vi "Acquisition & Generation (Init Memory-clock) test - Copia.vi"   [LabVIEW 2014]
uses:
  <vilib>/Platform/TimedLoop/XDataNode/timing_clust.ctl
  <vilib>/Platform/TimedLoop/XDataNode/nitl_modes.ctl
  <vilib>/Platform/TimedLoop/XDataNode/wakeup.ctl
  <vilib>/rvi/Emulation/niFpgaSctlEmulationGetInTimedLoop.vi
  <vilib>/rvi/Emulation/niFpgaEmulationReportErrorSimple.vi
  <vilib>/rvi/Emulation/niFpgaGetClockAttributes.vi
  <vilib>/rvi/Emulation/niFpgaCriticalErrorInLSC.vi
  <vilib>/rvi/Memory/Memory_Emulation/nirvimemoryFastEmulation.vi
  <vilib>/rvi/Memory/Memory_Emulation/nirvimemoryEmulation.vi
  <vilib>/rvi/Emulation/niFpgaEmulationIsFPGAContextNoSignature.vi
  <vilib>/rvi/DataTransferAndStorage/Container/Common/niFpgaContainerGetUniqueNameForEmu.vi
  <vilib>/rvi/Emulation/niFpgaProcessEmulError.vi
  <vilib>/rvi/errors/nirviReportUnexpectedCaseInternalError (U32).vi
  <vilib>/rvi/errors/niFpgaSetErrorForExecOnDevCompSimple.vi
  <vilib>/rvi/eio/common/nirviEmuReportErrorAndStop.vi
  <vilib>/rvi/FIFO/Fifo_Resource/nirvififoEmulationSetSize.vi
  <vilib>/rvi/FIFO/Fifo_Resource/nirviFifoEmulationQueueMgr.vi
  <instcachedir>/0/nirviFifoEmulationQueueMgr_E5CAEC123FF24DC58D834DCA3CDAA9B5.lvgen/nirviFifoEmulationQueueMgr_E5CAEC123FF24DC58D834DCA3CDAA9B5_010.vi
  <vilib>/rvi/FIFO/Fifo_Resource/nirvififoEmulationDetermineInputValidOut.vi
  <vilib>/rvi/FIFO/Fifo_Resource/nirvififoEmulationCreateLock.vi
  <vilib>/rvi/FIFO/Fifo_Resource/nirvififoEmulationObtainLock.vi
  <vilib>/rvi/FIFO/Fifo_Resource/nirvififoEmulationReleaseLock.vi
  <vilib>/rvi/occurrence/nirviWaitOnOccurrenceBase.vi
  <vilib>/rvi/errors/nirviReportUnexpectedCaseInternalError.vi
  <vilib>/rvi/eio/common/nirviEmuTemplateMethod_errors.vi
  <vilib>/rvi/interface/RandomDataEmulation/niFpgaRandomDataHandleErrors.vi
  <vilib>/Platform/TimedLoop/XDataNode/XDataNode.xnode
  <vilib>/rvi/DataTransferAndStorage/Container/XNode/niFpgaContainer.xnode
  <vilib>/rvi/FIFO/Fifo_Resource/nirvififoEmulationWrite.vi
  <vilib>/rvi/FIFO/Fifo_Resource/nirvififoEmulationRead.vi
  <vilib>/eio/EIOMethodNode/EIOMethodNode.xnode
  <vilib>/rvi/interface/RandomDataEmulation/nirviRandomDataFpgaReadWriteTemplate.vi
  <vilib>/Platform/TimedLoop/XDataNode/XDNodeRunTimeDep.lvlib
types:
  T1 = typedef "XDNodeRunTimeDep.lvlib/timing_clust.ctl" = cluster{"Expected End [f-1]":u64, "Actual End [f-1]":u64, "Finished Late? [f-1]":bool, "Expected End [i-1]":u64, "Actual End [i-1]":u64, "Finished Late? [i-1]":bool, "Expected Start [i]":u64, "Actual Start [i]":u64, "Expected Start [f]":u64, "Actual Start [f]":u64, "Source Name":string, "Structure Name":string, "Period":i64, "Deadline":i64, "Offset":i64, "Start":i64, "Priority":i32, "Timeout":i32, "Mode":T2, "Wakeup Reason":T3, "Error":errorcluster, "Source Type":string, "Secondary Source Type":string, "Global End Time":u64, "Global Start Time":u64, "Frame Duration":u64, "Iteration Duration":u64, "Assigned CPU":i32, "I/O Scan Engine Mode":u32}
  T2 = typedef "XDNodeRunTimeDep.lvlib/nitl_modes.ctl" = enum32{"No Change", "Process missed periods, maintain original phase", "Discard missed periods, maintain original phase", "Process missed periods, ignore original phase", "Discard missed periods, ignore original phase"}
  T3 = typedef "XDNodeRunTimeDep.lvlib/wakeup.ctl" = enum32{"Normal", "Aborted", "Asynchronous wakeup", "Timing source error", "Timed loop error", "Timeout"}
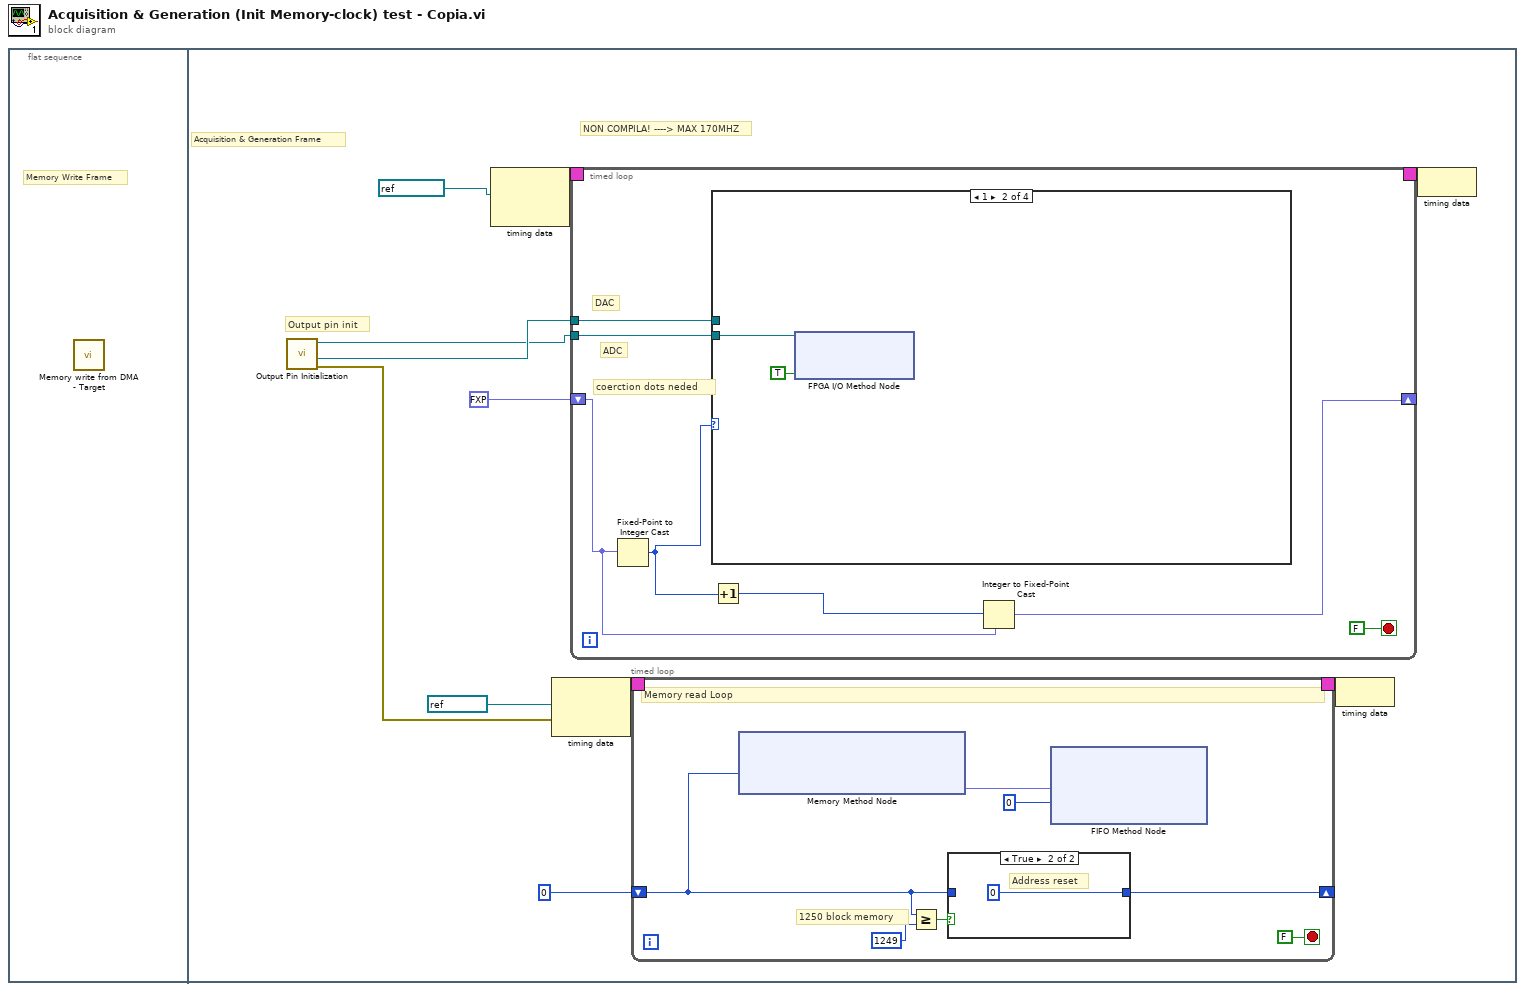
[diagram p0: block diagram]
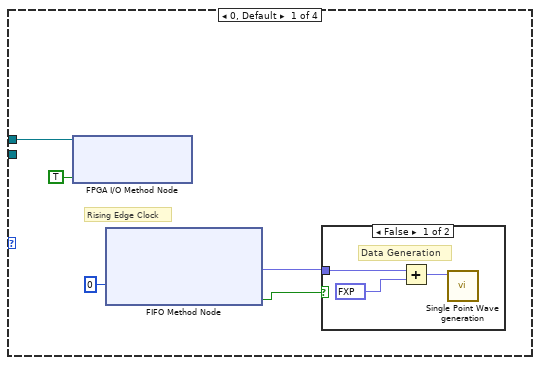
[diagram p2: hidden frame]
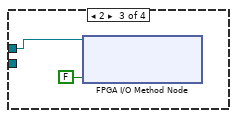
[diagram p4: hidden frame]
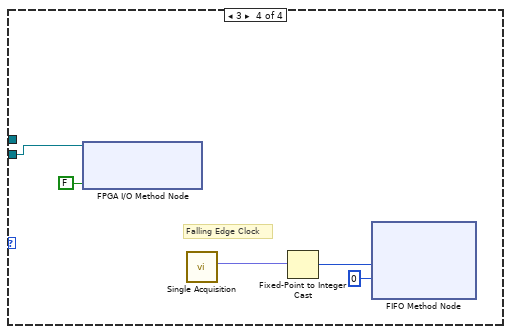
[diagram p5: hidden frame]
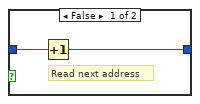
[diagram p6: hidden frame]
diagram:
  n1 = flat-sequence {
    frame #0 {
      # "Memory Write Frame"
      n2 = call "Memory write from DMA - Target.vi"() -> ()  [unwired: 12 in]
    }
    frame #1 {
      # "NON COMPILA! ----> MAX 170MHZ"
      # "Acquisition & Generation Frame"
      # "Output pin init"
      n3 = call "Output Pin Initialization.vi"() -> ("error out"=w7:errorcluster, "I/O Out Clock DAC (pin16)"=w3:refnum<k21>, "I/O Out Clock ADC (pin17)"=w2:refnum<k21>)  [unwired: 8 in]
      n4 = node-c288(refnum<k21> "200MHz" ("Source Name")) -> (w6:T1)  [unwired: 1 in]
      n5 = node-c288(refnum<k21> "50MHz" ("Source Name"), w7) -> (w11:T1)
      n6 = timed-loop {
        timing: w6 -> [_]
        timing-out: [_] -> w5
        shift-right: [w12] -> _
        shift-left: fxp<+,2,2> 0.0 -> [w13]
        tunnel: w3 -> [w17]
        tunnel: w2 -> [w16]
        stop <- FALSE stop-if-true
        # "ADC"
        # "DAC"
        # "coerction dots neded"
        n7 = Fixed-Point to Integer Cast(1:w13) -> (0:w15:u8)
        n8 = case shown="1" w15 {
          tunnel: w17 -> [w23 _ w30 _]
          tunnel: w16 -> [_ w28 _ w35]
          frame 0, Default {
            # "Rising Edge Clock"
            n9 = xnode "FPGA I/O Method Node"("FPGA I/O In"=w23, "Data"=TRUE) -> ()  [unwired: 1 out]
            n10 = xnode ("FIFO Method Node")("Timeout"=0) -> ("Element"=w19:fxp<+/-,12,12>, "Timed Out?"=w20:bool)  [unwired: 1 in, 1 out]
            n11 = case shown="False" w20 {
              tunnel: w19 -> [w26 _]
              frame False {
                # "Data Generation"
                n12 = Add(x=w26, y=fxp<+,12,12> 2048.0) -> (x+y=w24:fxp<+/-,14,14>)
                n13 = call "Single Point Wave generation.vi"("Data To Write"=w24) -> ()  [unwired: 10 in, 1 out]
              }
              frame True {
                # "FPGA memory slow"
              }
            }
          }
          frame 1 {
            n14 = xnode "FPGA I/O Method Node"("FPGA I/O In"=w28, "Data"=TRUE) -> ()  [unwired: 1 out]
          }
          frame 2 {
            n15 = xnode "FPGA I/O Method Node"("FPGA I/O In"=w30, "Data"=FALSE) -> ()  [unwired: 1 out]
          }
          frame 3 {
            # "Falling Edge Clock"
            n16 = xnode "FPGA I/O Method Node"("FPGA I/O In"=w35, "Data"=FALSE) -> ()  [unwired: 1 out]
            n17 = call "Single Acquisition.vi"() -> ("Out"=w31:fxp<+/-,12,12>)  [unwired: 10 in, 1 out]
            n18 = Fixed-Point to Integer Cast(1:w31) -> (0:w32:i16)
            n19 = xnode ("FIFO Method Node")("Element"=w32, "Timeout"=0) -> ()  [unwired: 1 in, 2 out]
          }
        }
        n20 = Increment(x=w15) -> (x+1=w14:u8)
        n21 = Integer to Fixed-Point Cast(fixed-point type=w13, integer=w14) -> (fixed-point=w12:fxp<+,2,2>)
      }
      n22 = timed-loop {
        timing: w11 -> [_]
        timing-out: [_] -> w10
        shift-right: [w46] -> _
        shift-left: u32 0 -> [w44]
        stop <- FALSE stop-if-true
        # "1250 block memory"
        # "Memory read Loop"
        n23 = xnode ("Memory Method Node")("Address"=w44) -> ("Data"=w43:fxp<+/-,12,12>)  [unwired: 1 in, 1 out]
        n24 = Greater Or Equal?(x=w44, y=u32 1249) -> (x >= y?=w47:bool)
        n25 = case shown="True" w47 {
          tunnel: w44 -> [w50 _]
          tunnel: [w49 u32 0] -> w46
          frame False {
            # "Read next address"
            n26 = Increment(x=w50) -> (x+1=w49:u32)
          }
          frame True {
            # "Address reset"
          }
        }
        n27 = xnode ("FIFO Method Node")("Element"=w43, "Timeout"=0) -> ()  [unwired: 1 in, 2 out]
      }
      n28 = node-c288(w10) -> ()
      n29 = node-c288(w5) -> ()
    }
  }
